vi "CIC_stage.vi"(8 "decimate factor":i16, 9 "New Data":bool, 11 "input":i64) -> (1 "Data Ready":bool, 3 "output":i64)   [LabVIEW 2009]
panel:
  in  "count":i16
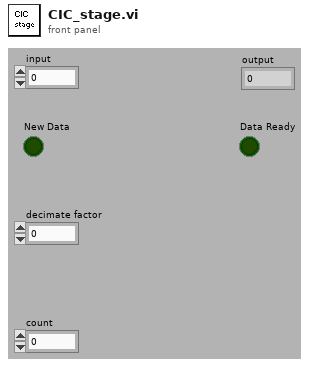
[diagram p1: front panel]
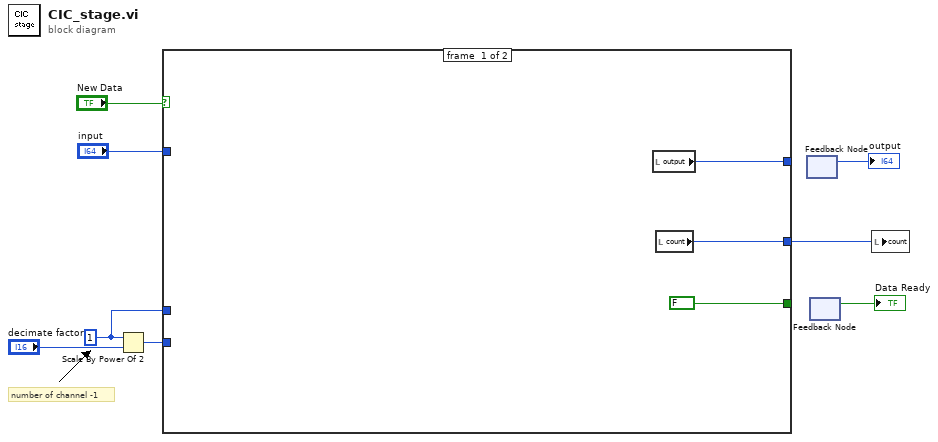
[diagram p0: block diagram]
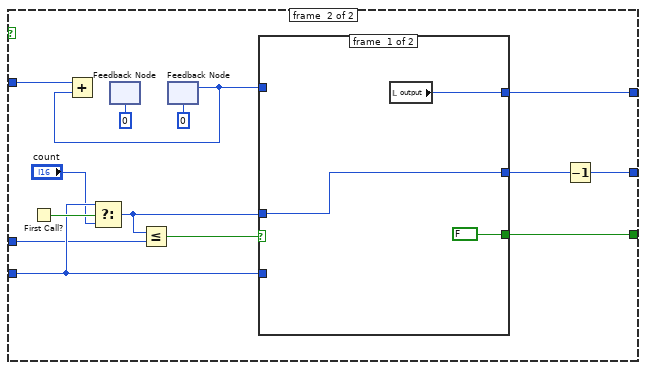
[diagram p2: hidden frame]
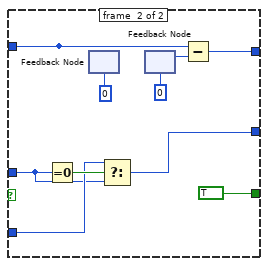
[diagram p3: hidden frame]
diagram:
  w1 = 1 ("n")
  # "number of channel -1"
  n1 = Scale By Power Of 2(n=w1, x="decimate factor") -> (x*2^n=w2:i16)
  n2 = case shown="True" "New Data" {
    tunnel: [w12 w29] -> w7
    tunnel: w2 -> [_ w18]
    tunnel: [w13 w27] -> w10
    tunnel: "input" -> [_ w25]
    tunnel: [FALSE ("Data Ready") w24] -> w5
    tunnel: w1 -> [_ w14]
    frame #0 {
      n3 = local read "output"() -> (w12:i64)
      n4 = local read "count"() -> (w13:i16)
    }
    frame #1 {
      n5 = First Call?() -> (First Call?: T/F=w19:bool)
      n6 = Select(t=w18, s=w19, f="count") -> (s? t:f=w15:i16)
      n7 = feedback #1(i64 0) -> (w22:i64)
      n8 = Less Or Equal?(x=w15, y=w14) -> (x <= y?=w16:bool)
      n9 = feedback #2(i64 0) -> (w21:i64)
      n10 = Add(x=w25, y=w21) -> (x+y=w23:i64)
      n11 = case shown="True" w16 {
        tunnel: w21 -> [_ w38]
        tunnel: [w32 w40] -> w29
        tunnel: [w30 w33] -> w28
        tunnel: w18 -> [_ w35]
        tunnel: [FALSE ("Data Ready") TRUE ("Data Ready")] -> w24
        tunnel: w15 -> [w30 w34]
        frame #0 {
          n12 = local read "output"() -> (w32:i64)
        }
        frame #1 {
          n13 = Equal To 0?(x=w34) -> (x = 0?=w36:bool)
          n14 = feedback #3(i64 0) -> (w39:i64)
          n15 = Select(t=w35, s=w36, f=w34) -> (s? t:f=w33:i16)
          n16 = feedback #4(i64 0) -> (w43:i64)
          n17 = Subtract(x=w38, y=w43) -> (x-y=w40:i64)
        }
      }
      n18 = Decrement(x=w28) -> (x-1=w27:i16)
    }
  }
  n19 = feedback #5() -> (→"output":i64)  [unwired: 1 out]
  n20 = feedback #6() -> (→"Data Ready":bool)  [unwired: 1 out]
  n21 = local write "count"(w10) -> ()
